vi "Supplementary Angle.vi"   [LabVIEW 2017, in "NI_AAL_Angle.lvlib"]
doc: "Calculates the supplementary angle of the input angle.\n\nWire data to any of the angle inputs to determine the polymorphic instance to use or manually select the instance."
uses:
  <vilib>/Analysis/NI_AAL_Angle.lvlib
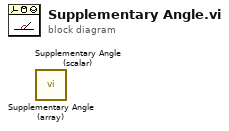
[diagram p0: block diagram]
diagram:
  n1 = call <vilib>:"Supplementary Angle (array).vi"() -> ()  [unwired: 10 in, 2 out]
  n2 = call <vilib>:"Supplementary Angle (scalar).vi"() -> ()  [unwired: 10 in, 2 out]
